vi "hpcnc construct and send gcode.vi"(8 "error in (no error)":errorcluster, 10 "GCode":string, 11 "VISA Refnum in":refnum<visa-resource-name>) -> (0 "error out":errorcluster, 3 "VISA Refnum out":refnum<visa-resource-name>)   [LabVIEW 2014]
uses:
  HPCNC.lvlib
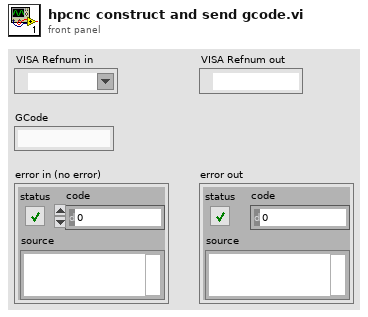
[diagram p1: front panel]
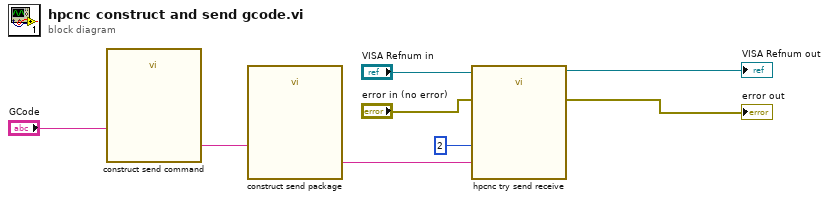
[diagram p0: block diagram]
diagram:
  n1 = call "construct send command.vi"("GCode"="GCode") -> ("SendCommand"=w8:string)  [unwired: 9 in]
  n2 = call "construct send package.vi"("Send command"=w8) -> ("Send package"=w5:string)  [unwired: 8 in, 2 out]
  n3 = call "hpcnc try send receive.vi"("error in (no error)"="error in (no error)", "Max try number"=2, "Send package"=w5, "VISA Refnum in"="VISA Refnum in") -> ("error out"=→"error out":errorcluster, "VISA Refnum out"=→"VISA Refnum out":refnum<visa-resource-name>)  [unwired: 4 in, 2 out]
